vi "LvHostsEdit4cRIO_SUB_HostEdit_Dialog.vi"(10 "HostInfo":T1) -> (1 "Cancel?":bool, 2 "HostInfo out":T1)   [LabVIEW 2014]
uses:
  LvHostsEdit4cRIO_Rsc_HostInfo_Typedef.ctl
panel:
  in  "Btn Cancel":bool
  in  "Btn OK":bool
  in  "Coment":string
  in  "Alias":string
  in  "Hostname":string
  in  "IP Address":string
  in  "enable":bool
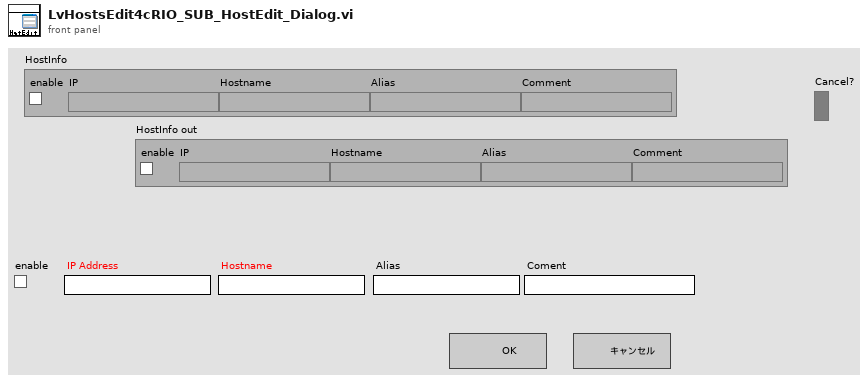
[diagram p1: front panel]
types:
  T1 = typedef "LvHostsEdit4cRIO_Rsc_HostInfo_Typedef.ctl" = cluster{"enable":bool, "IP":string, "Hostname":string, "Alias":string, "Comment":string}
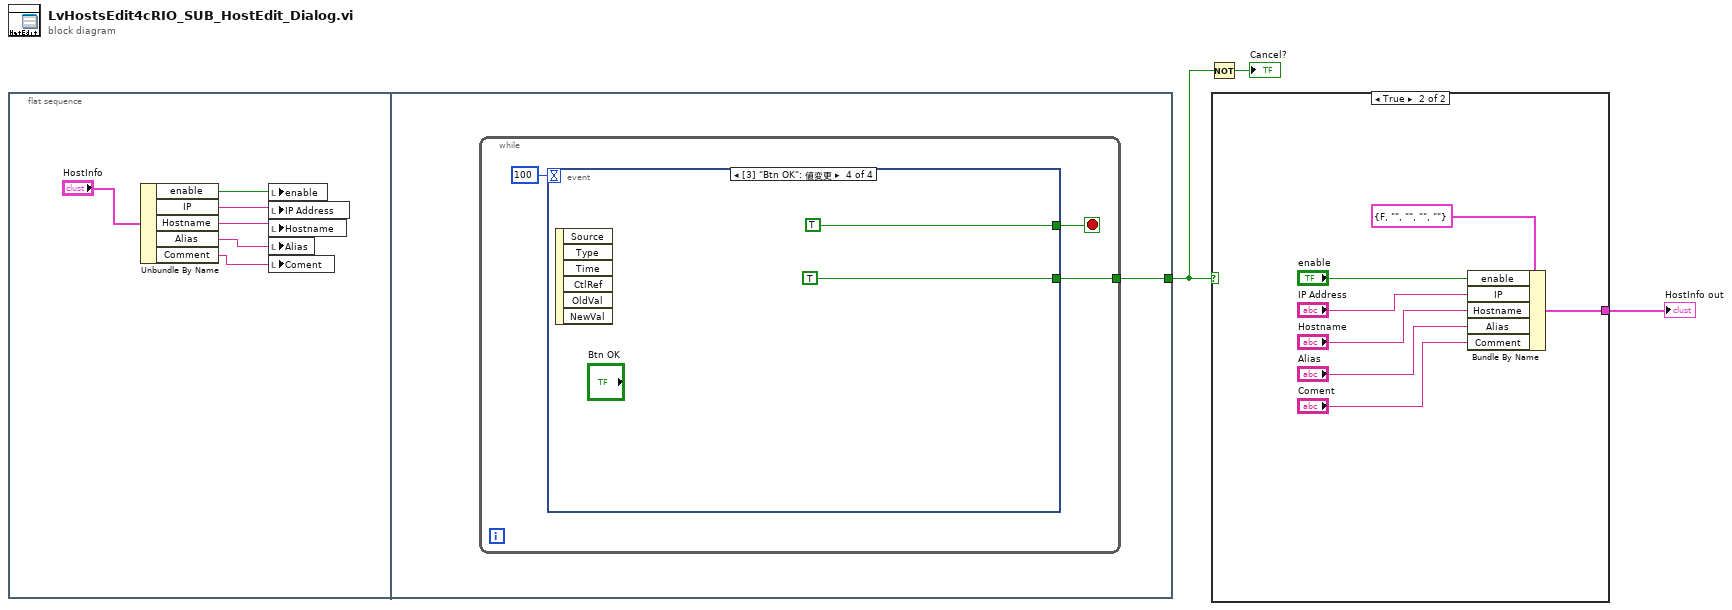
[diagram p0: block diagram]
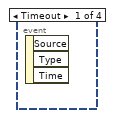
[diagram p3: hidden frame]
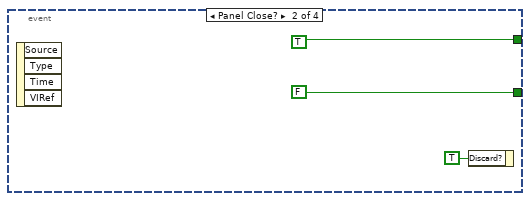
[diagram p4: hidden frame]
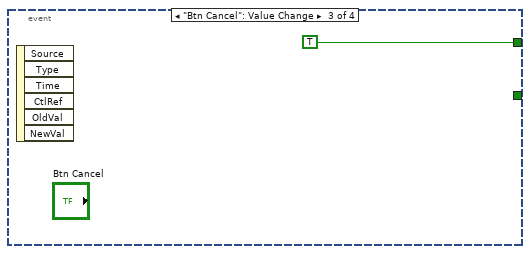
[diagram p5: hidden frame]
diagram:
  n1 = flat-sequence {
    tunnel: [w10] -> w3
    frame #0 {
      n2 = Unbundle By Name("HostInfo") -> ("enable"=w8:bool, "IP"=w7:string, "Hostname"=w6:string, "Alias"=w5:string, "Comment"=w4:string)
      n3 = local write "enable"(w8) -> ()
      n4 = local write "IP Address"(w7) -> ()
      n5 = local write "Hostname"(w6) -> ()
      n6 = local write "Alias"(w5) -> ()
      n7 = local write "Coment"(w4) -> ()
    }
    frame #1 {
      n8 = while {
        tunnel: [w11] -> w10
        stop <- w12 stop-if-true
        n9 = event shown="[3] \"Btn OK\": 値変更" {
          selector: _ -> [_ _ _ _]
          dyn-events: _ -> [_ _ _ _]
          timeout: 100 -> [_ _ _ _]
          tunnel: [_ TRUE TRUE TRUE] -> w12
          tunnel: [_ FALSE _ TRUE] -> w11
          event Timeout {
            n10 = event-data() -> ()  [unwired: 1 in, 3 out]
          }
          event Panel Close? {
            n11 = event-data() -> ()  [unwired: 1 in, 4 out]
            n12 = event-data("Discard?"=TRUE ("破棄?")) -> ()  [unwired: 1 in, 1 out]
          }
          event "Btn Cancel": Value Change {
            n13 = event-data() -> ()  [unwired: 1 in, 6 out]
          }
          event "Btn OK": Value Change {
            n14 = event-data() -> ()  [unwired: 1 in, 6 out]
          }
        }
      }
    }
  }
  n15 = Not(x=w3) -> (.not. x?=→"Cancel?":bool)
  n16 = case shown="TRUE" w3 {
    tunnel: [_ w24] -> w1
    frame False {
      # "Cancel"
    }
    frame True {
      n17 = Bundle By Name(cluster=T1 {"enable"=FALSE, "IP"="", "Hostname"="", "Alias"="", "Comment"=""} ("HostInfo out"), "enable"="enable", "IP"="IP Address", "Hostname"="Hostname", "Alias"="Alias", "Comment"="Coment") -> (w24:T1)
    }
  }
  "HostInfo out" <- w1
